vi "Priority Enqueue.vi"(8 "error in (no error)":errorcluster, 9 "Message":refnum<class "Message.lvclass">, 10 "Priority":i32, 11 "Priority Message Queue in":refnum<class "Priority Message Queue.lvclass">) -> (0 "error out":errorcluster, 3 "Priority Message Queue out":refnum<class "Priority Message Queue.lvclass">)   [LabVIEW 2022 SP3, in "Artifex.lvlib" / "Priority Message Queue.lvclass"]
uses:
  Priority Message Queue.lvclass
  Priority Message Queue.lvclass/Priority Message Queue.ctl
  Message/Message.lvclass
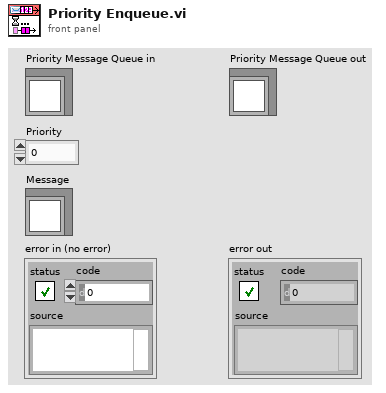
[diagram p1: front panel]
types:
  T1 = typedef "Artifex.lvlib/Priority Message Queue.lvclass/Ref Data.ctl" = cluster{"# Waiting":u32, "Buffers":refnum<queue>[], "Wait Msg":refnum<queue>, "Wait Prior":refnum<queue>}
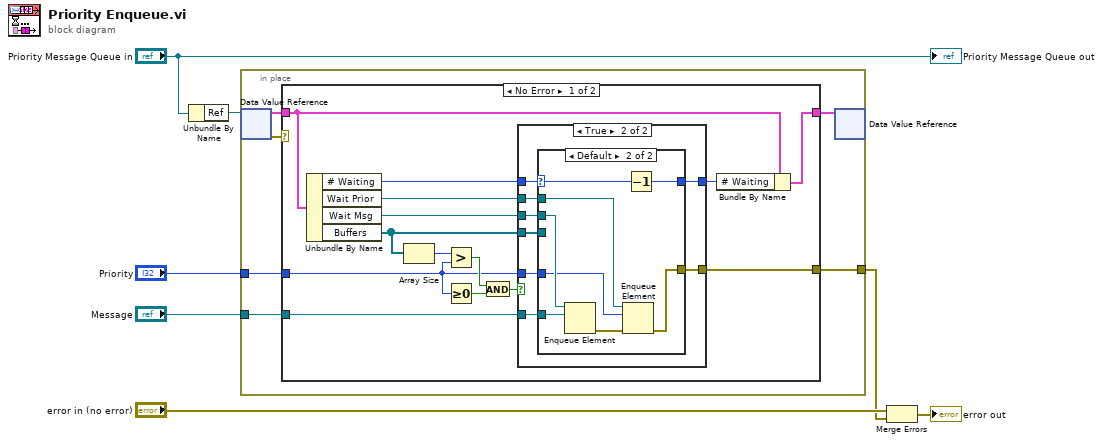
[diagram p0: block diagram]
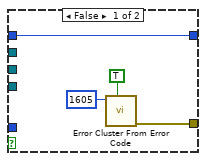
[diagram p2: hidden frame]
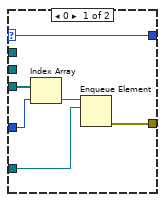
[diagram p3: hidden frame]
diagram:
  n1 = Unbundle By Name("Priority Message Queue in") -> ("Ref"=w5:refnum<data-value>)
  n2 = in-place {
    in-place-border: "Priority" -> [w11]
    in-place-border: "Message" -> [w10]
    in-place-border: [w9] -> w1
    n3 = in-place-dvr #1(w5) -> (w12:T1, w13:errorcluster)
    n4 = case shown="No Error" w13 {
      selector: w13 -> [_ w54]
      tunnel: w12 -> [w16 w55]
      tunnel: w11 -> [w22 _]
      tunnel: w10 -> [w23 _]
      tunnel: [w21 w54] -> w9
      tunnel: [w14 w55] -> w8
      frame No Error {
        n5 = Unbundle By Name(w16) -> ("# Waiting"=w20:u32, "Wait Prior"=w19:refnum<queue>, "Wait Msg"=w18:refnum<queue>, "Buffers"=w17:refnum<queue>[])
        n6 = Array Size(array=w17) -> (size(s)=w27:i32)
        n7 = Greater?(x=w27, y=w22) -> (0:w26:bool)
        n8 = Greater Or Equal To 0?(x=w22) -> (x >= 0?=w25:bool)
        n9 = And(x=w26, y=w25) -> (x .and. y?=w24:bool)
        n10 = case shown="True" w24 {
          tunnel: w23 -> [_ w36]
          tunnel: w22 -> [_ w35]
          tunnel: [w29 w34] -> w21
          tunnel: w20 -> [w28 w39]
          tunnel: w19 -> [_ w38]
          tunnel: w18 -> [_ w37]
          tunnel: [w28 w33] -> w15
          tunnel: w17 -> [_ w32]
          frame False {
            n11 = call <vilib>:"Error Cluster From Error Code.vi"("show call chain? (False)"=TRUE, "error code (0)"=1605) -> ("error out"=w29:errorcluster)  [unwired: 7 in]
          }
          frame True {
            n12 = case shown="Default" w39 {
              selector: w39 -> [w40 w53]
              tunnel: w38 -> [_ w49]
              tunnel: w37 -> [_ w50]
              tunnel: w36 -> [w42 w52]
              tunnel: w35 -> [w44 w48]
              tunnel: [w41 w47] -> w34
              tunnel: [w40 w46] -> w33
              tunnel: w32 -> [w45 _]
              frame 0 {
                n13 = Index Array(array=w45, index=w44) -> (element=w43:refnum<queue>)
                n14 = Enqueue Element(queue=w43, element=w42) -> (error out=w41:errorcluster)  [unwired: 2 in, 2 out]
              }
              frame Default {
                n15 = Enqueue Element(queue=w50, element=w52) -> (error out=w51:errorcluster)  [unwired: 2 in, 2 out]
                n16 = Enqueue Element(queue=w49, element=w48, error in (no error)=w51) -> (error out=w47:errorcluster)  [unwired: 1 in, 2 out]
                n17 = Decrement(x=w53) -> (x-1=w46:u32)
              }
            }
          }
        }
        n18 = Bundle By Name(cluster=w16, "# Waiting"=w15) -> (w14:T1)
      }
      frame Error {
      }
    }
    n19 = in-place-dvr #1(w8) -> ()  [unwired: 2 out]
  }
  n20 = Merge Errors("error in (no error)", w1) -> (→"error out":errorcluster)
  "Priority Message Queue out" <- "Priority Message Queue in"
